vi "Channel ctrl disabled synergy-Bgnd MovCor.vi"(8 "error in (no error)":errorcluster, 11 "Behaviour":T1) -> (0 "error out":errorcluster)   [LabVIEW 2017]
uses:
  Typedefs/Channel control synergistic behaviour enum.ctl
  Globals/gl_Windows Ctrl refs.vi
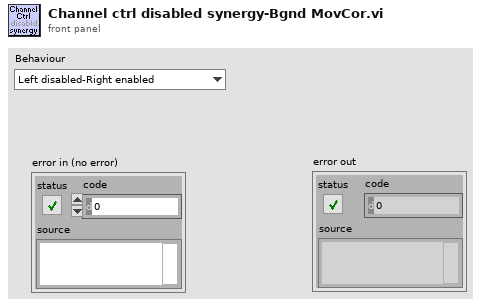
[diagram p1: front panel]
types:
  T1 = typedef "Channel control synergistic behaviour enum.ctl" = enum16{"Left disabled-Right enabled", "Left enabled-Right disabled", "Both enabled"}
  T2 = typedef "Live window-ctrl refs.ctl" = cluster{"This VI":refnum<vi>, "Pane":refnum<vi>, "Show REF Image Left":refnum<vi>, "Show REF Image Right":refnum<vi>, "Snapshot":refnum<vi>, "Left Image Palette":refnum<vi>, "Right Image Palette":refnum<vi>, "Left Channel":refnum<vi>, "Right Channel":refnum<vi>, "Left image intensity":refnum<vi>, "Right image intensity":refnum<vi>, "Left Image Display":T3, "Right Image Display":T3, "Refresh rate ind (Hz)":refnum<vi>, "Acq rate ind (Hz)":refnum<vi>, "Stop (ind)":refnum<vi>}
  T3 = typedef "Image display ref.ctl" = refnum<vi>
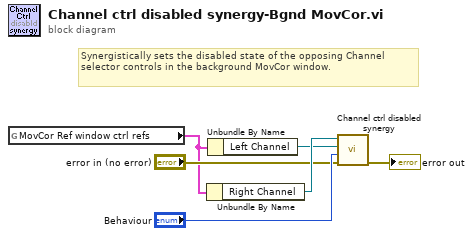
[diagram p0: block diagram]
diagram:
  # "Synergistically sets the disabled state of the opposing Channel selector controls in the background MovCor window."
  n1 = global read "gl_Windows Ctrl refs.vi" "MovCor Ref window ctrl refs"() -> (w1:T2)
  n2 = Unbundle By Name(w1) -> ("Right Channel"=w5:refnum<vi>)
  n3 = Unbundle By Name(w1) -> ("Left Channel"=w4:refnum<vi>)
  n4 = call "Channel ctrl disabled synergy.vi"("error in (no error)"="error in (no error)", "Behaviour"="Behaviour", "Right Channel"=w4, "Left Channel"=w5) -> ("error out"=→"error out":errorcluster)  [unwired: 7 in]
